vi "JAPsubscribeBOOL(NI).vi"(8 "error in (no error)":errorcluster, 11 "JAPCboolIN":refnum<class "JSubscribe.lvclass">) -> (0 "error out":errorcluster, 2 "JAPCbool":string, 3 "JAPCboolOUT":refnum<class "JSubscribe.lvclass">)   [LabVIEW 2014]
uses:
  <userlib>/_RADE/RIO/JAPC/classes/JSubscribe/JSubscribe.lvclass
  <userlib>/_RADE/RIO/JAPC/classes/JSubscribe/JAPCSubscribe.vi
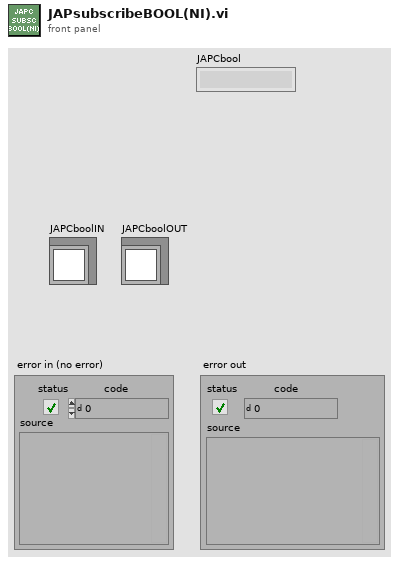
[diagram p1: front panel]
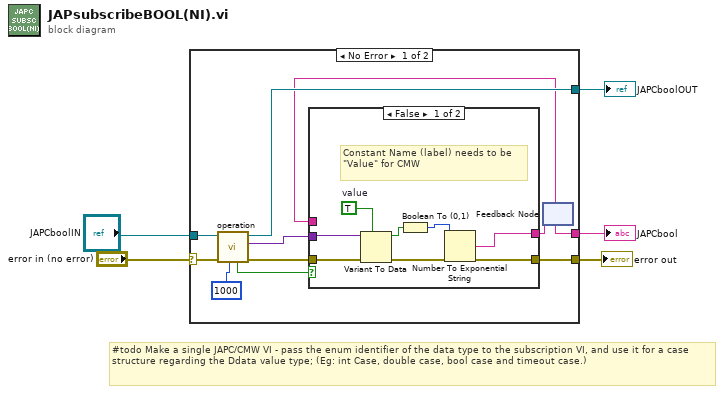
[diagram p0: block diagram]
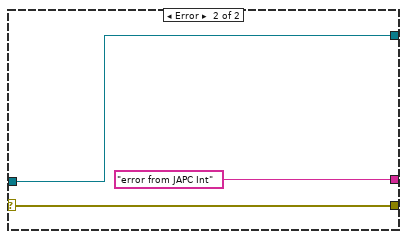
[diagram p3: hidden frame]
diagram:
  # "#todo Make a single JAPC/CMW VI - pass the enum identifier of the data type to the subscription VI, and use it for a case structure regarding the Ddata value type; (Eg: int Case, double case, bool case and timeout case.)"
  n1 = case shown="No Error" "error in (no error)" {
    selector: "error in (no error)" -> [w10 w27]
    tunnel: [w14 w27] -> w1
    tunnel: "JAPCboolIN" -> [w11 w26]
    tunnel: [w8 w26] -> w2
    tunnel: [w6 "error from JAPC Int"] -> w3
    frame No Error {
      n2 = call-poly <userlib>:"operation.vi"("Timeout (10000 ms)"=1000, "error in (no error)"=w10, "Object in"=w11) -> ("error out"=w15:errorcluster, "Data"=w9:variant, "Object out"=w8:refnum<class "JSubscribe.lvclass">, "Timeout?"=w12:bool)  [unwired: 3 in, 2 out]
      n3 = feedback #1() -> (w6:string)  [unwired: 1 in]
      n4 = case shown="False" w12 {
        tunnel: w15 -> [w22 w24]
        tunnel: [w20 w24] -> w14
        tunnel: w9 -> [w21 _]
        tunnel: [w19 w23] -> w7
        tunnel: w6 -> [_ w23]
        frame False {
          w18 = TRUE  # value
          # "Constant Name (label) needs to be \"Value\" for CMW"
          n5 = Variant To Data(error in=w22, type=w18, Variant=w21) -> (data=w16:bool, error out=w20:errorcluster)
          n6 = Boolean To (0,1)(Boolean=w16) -> (0, 1=w17:i16)
          n7 = Number To Exponential String(number=w17) -> (E-format string=w19:string)  [unwired: 3 in]
        }
        frame True {
          # "Subscription Timed Out"
        }
      }
      n8 = feedback-in #1(w7) -> ()
    }
    frame Error {
    }
  }
  "error out" <- w1
  "JAPCboolOUT" <- w2
  "JAPCbool" <- w3
